vi "AssertControlValueUntillTrue.vi"(0 "VI Reference In":refnum<vi>, 1 "Label":string, 5 "Control Name":string, 7 "Control Value":variant, 9 "Timeout(5 sec)":dbl=5.0, 11 "error out":errorcluster, 12 "Compare":T1) -> (4 "VI Reference Out":refnum<vi>, 15 "error out":errorcluster)   [LabVIEW 2016]
doc: "<b>This VI asserts the value of controls in other VI.<b> \n\nThe input control name is given as a string , incase of path, use delimiters inbetween the path.\nThis VI gets the value of the control, untill the value is equal to the input value."
uses:
  TypeDef/ComparisionTypeControl.ctl
  AssertControlValueByPathString.vi
  <vilib>/addons/_JKI Toolkits/Caraya/classes/Assert/Assert Equal Value and Type_Variant.vi
  <vilib>/addons/_JKI Toolkits/Caraya/classes/Assert/Assert Not Equal Value and Type_Variant.vi
  <vilib>/addons/_JKI Toolkits/Caraya/classes/Assert/Assert Greater_Variant.vi
  <vilib>/addons/_JKI Toolkits/Caraya/classes/Assert/Assert Greater Or Equal_Variant.vi
  <vilib>/addons/_JKI Toolkits/Caraya/classes/Assert/Assert Less_Variant.vi
  <vilib>/addons/_JKI Toolkits/Caraya/classes/Assert/Assert Less Or Equal_Variant.vi
  <vilib>/addons/_JKI Toolkits/Caraya/classes/Assert/Assert.lvclass
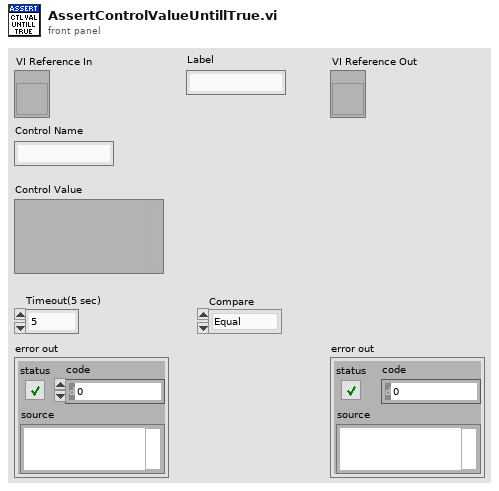
[diagram p1: front panel]
types:
  T1 = typedef "ComparisionTypeControl.ctl" = enum16{"Equal", "Not Equal", "Greater", "Greater or Equal", "Lesser", "Lesser or Equal"}
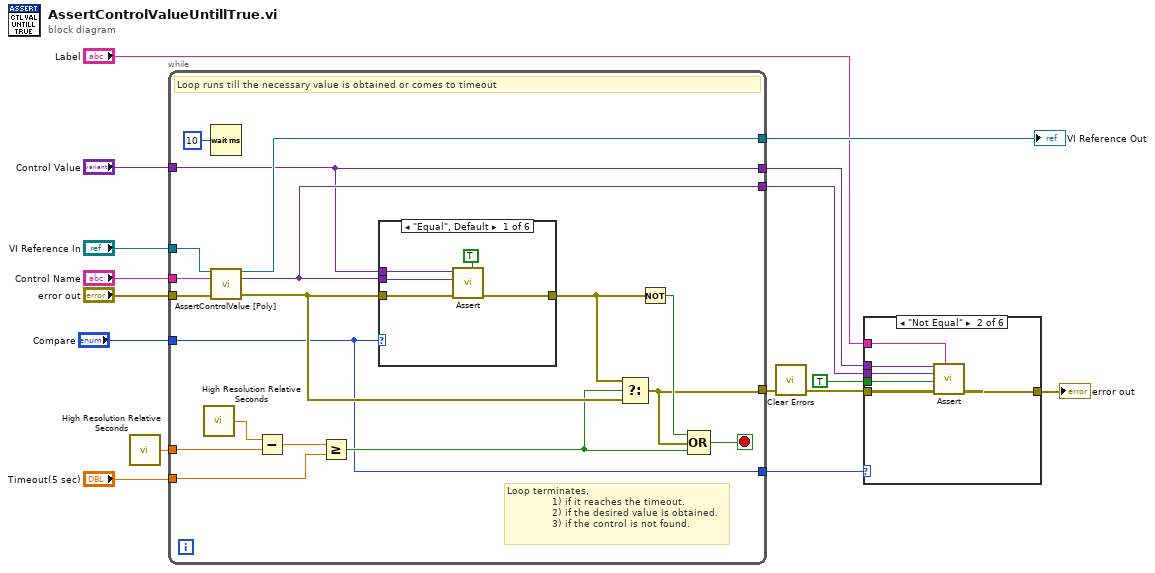
[diagram p0: block diagram]
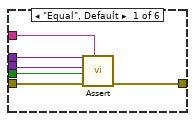
[diagram p2: hidden frame]
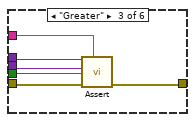
[diagram p3: hidden frame]
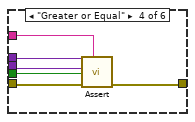
[diagram p4: hidden frame]
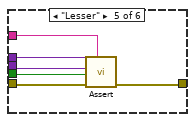
[diagram p5: hidden frame]
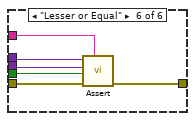
[diagram p6: hidden frame]
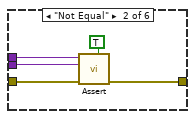
[diagram p7: hidden frame]
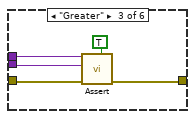
[diagram p8: hidden frame]
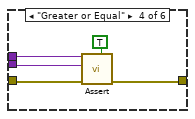
[diagram p9: hidden frame]
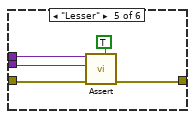
[diagram p10: hidden frame]
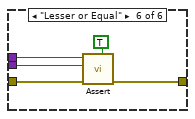
[diagram p11: hidden frame]
diagram:
  n1 = call <vilib>:"High Resolution Relative Seconds.vi"() -> ("relative seconds"=w13:dbl)
  n2 = while {
    tunnel: "Control Name" -> [w33]
    tunnel: "VI Reference In" -> [w32]
    tunnel: "Control Value" -> [w21]
    tunnel: "Timeout(5 sec)" -> [w26]
    tunnel: [w29] -> w10
    tunnel: w13 -> [w31]
    tunnel: "error out" -> [w34]
    tunnel: [w18] -> w9
    tunnel: [w21] -> w5
    tunnel: [w22] -> w4
    tunnel: "Compare" -> [w17]
    tunnel: [w17] -> w1
    stop <- w24 stop-if-true
    # "Loop terminates,\n               1) if it reaches the timeout.\n               2) if the desired value is obtained.\n               3) if the control is not found."
    # "Loop runs till the necessary value is obtained or comes to timeout"
    n3 = call <vilib>:"High Resolution Relative Seconds.vi"() -> ("relative seconds"=w30:dbl)
    n4 = Wait (ms)(milliseconds to wait=u32 10) -> ()  [unwired: 1 out]
    n5 = call-poly "AssertControlValue [Poly].vi"("VI Reference In"=w32, "Control Name"=w33, "error in"=w34) -> ("VI Reference Out"=w29:refnum<vi>, "Value"=w22:variant, "error out"=w25:errorcluster)  [unwired: 10 in]
    n6 = Subtract(x=w30, y=w31) -> (x-y=w27:dbl)
    n7 = Greater Or Equal?(x=w27, y=w26) -> (x >= y?=w20:bool)
    n8 = case shown="\"Equal\", Default" w17 {
      tunnel: w25 -> [w37 w43 w47 w52 w57 w62]
      tunnel: [w38 w42 w48 w53 w58 w63] -> w23
      tunnel: w22 -> [w35 w41 w45 w50 w55 w60]
      tunnel: w21 -> [w36 w40 w46 w51 w56 w61]
      frame "Equal", Default {
        n9 = call-poly <vilib>:"Assert.vi"("Assert Only? (F)"=TRUE, "error in (no error)"=w37, "Y"=w35, "X"=w36) -> ("error out"=w38:errorcluster)  [unwired: 7 in]
      }
      frame "Not Equal" {
        n10 = call-poly <vilib>:"Assert.vi"("Assert Only? (F)"=TRUE, "error in (no error)"=w43, "Y"=w41, "X"=w40) -> ("error out"=w42:errorcluster)  [unwired: 7 in]
      }
      frame "Greater" {
        n11 = call-poly <vilib>:"Assert.vi"("Assert Only? (F)"=TRUE, "error in (no error)"=w47, "Y"=w45, "X"=w46) -> ("error out"=w48:errorcluster)  [unwired: 7 in]
      }
      frame "Greater or Equal" {
        n12 = call-poly <vilib>:"Assert.vi"("Assert Only? (F)"=TRUE, "error in (no error)"=w52, "Y"=w50, "X"=w51) -> ("error out"=w53:errorcluster)  [unwired: 7 in]
      }
      frame "Lesser" {
        n13 = call-poly <vilib>:"Assert.vi"("Assert Only? (F)"=TRUE, "error in (no error)"=w57, "Y"=w55, "X"=w56) -> ("error out"=w58:errorcluster)  [unwired: 7 in]
      }
      frame "Lesser or Equal" {
        n14 = call-poly <vilib>:"Assert.vi"("Assert Only? (F)"=TRUE, "error in (no error)"=w62, "Y"=w60, "X"=w61) -> ("error out"=w63:errorcluster)  [unwired: 7 in]
      }
    }
    n15 = Select(t=w23, s=w20, f=w25) -> (s? t:f=w18:errorcluster)
    n16 = Not(x=w23) -> (.not. x?=w19:bool)
    n17 = Compound Arithmetic op=OR(w19, w18, w20) -> (w24:bool)
  }
  "VI Reference Out" <- w10
  n18 = call <vilib>:"Clear Errors.vi"("error in (no error)"=w9) -> ("error out"=w7:errorcluster)  [unwired: 5 in, 1 out]
  n19 = case shown="\"Not Equal\"" w1 {
    tunnel: w7 -> [w69 w76 w81 w87 w93 w99]
    tunnel: [w70 w75 w82 w88 w94 w100] -> w6
    tunnel: w4 -> [w68 w74 w79 w85 w91 w97]
    tunnel: w5 -> [w66 w73 w80 w86 w92 w98]
    tunnel: TRUE ("Register with caller test (F)") -> [w67 w72 w78 w84 w90 w96]
    tunnel: "Label" -> [w65 w71 w77 w83 w89 w95]
    frame "Equal", Default {
      n20 = call-poly <vilib>:"Assert.vi"("Label"=w65, "error in (no error)"=w69, "Register with caller test (F)"=w67, "Y"=w68, "X"=w66) -> ("error out"=w70:errorcluster)  [unwired: 6 in]
    }
    frame "Not Equal" {
      n21 = call-poly <vilib>:"Assert.vi"("Label"=w71, "error in (no error)"=w76, "Register with caller test (F)"=w72, "Y"=w74, "X"=w73) -> ("error out"=w75:errorcluster)  [unwired: 6 in]
    }
    frame "Greater" {
      n22 = call-poly <vilib>:"Assert.vi"("Label"=w77, "error in (no error)"=w81, "Register with caller test (F)"=w78, "Y"=w79, "X"=w80) -> ("error out"=w82:errorcluster)  [unwired: 6 in]
    }
    frame "Greater or Equal" {
      n23 = call-poly <vilib>:"Assert.vi"("Label"=w83, "error in (no error)"=w87, "Register with caller test (F)"=w84, "Y"=w85, "X"=w86) -> ("error out"=w88:errorcluster)  [unwired: 6 in]
    }
    frame "Lesser" {
      n24 = call-poly <vilib>:"Assert.vi"("Label"=w89, "error in (no error)"=w93, "Register with caller test (F)"=w90, "Y"=w91, "X"=w92) -> ("error out"=w94:errorcluster)  [unwired: 6 in]
    }
    frame "Lesser or Equal" {
      n25 = call-poly <vilib>:"Assert.vi"("Label"=w95, "error in (no error)"=w99, "Register with caller test (F)"=w96, "Y"=w97, "X"=w98) -> ("error out"=w100:errorcluster)  [unwired: 6 in]
    }
  }
  "error out" <- w6
